vi "Parse Excel Doc.vi"(8 "error in (no error)":errorcluster, 11 "path":path) -> (0 "error out":errorcluster, 3 "Data":variant[][](array[variant]))   [LabVIEW 2019, in "Simple SysDef API.lvlib"]
uses:
  <userlib>/SimpleSysDef/Simple SysDef API.lvlib
panel:
  in  "Excel._Worksheet":refnum<k7>
  in  "Excel._Application":refnum<k7>
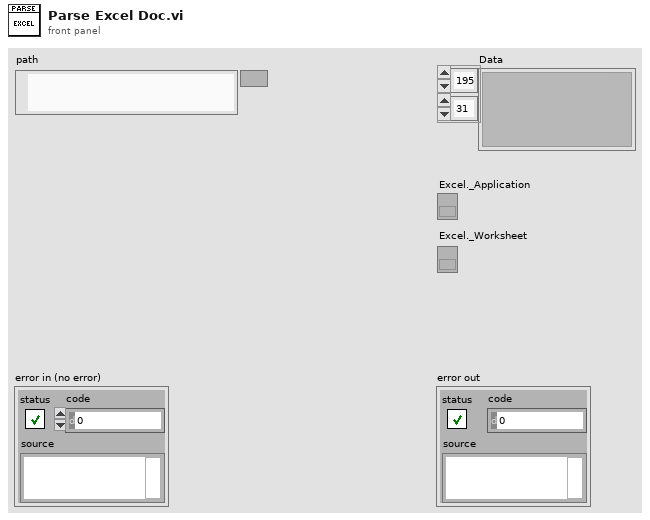
[diagram p1: front panel]
types:
  T1 = enum16{"maximized", "minimized", "normal", "no change"}
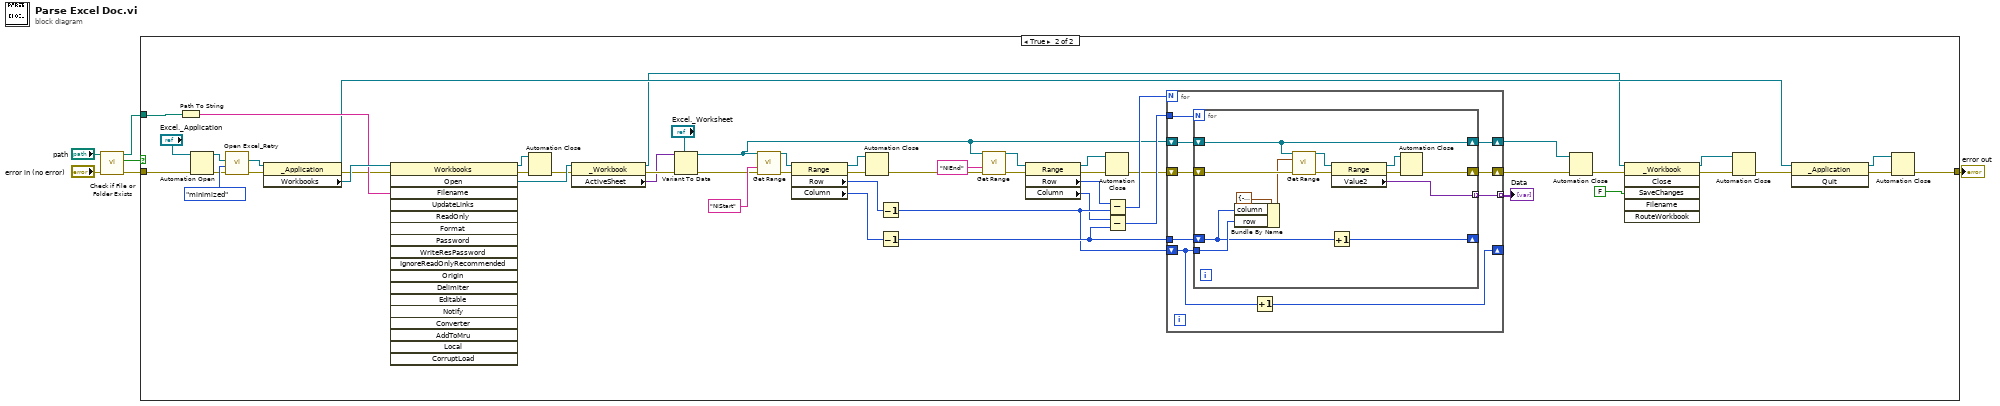
[diagram p0: block diagram]
diagram:
  n1 = call <vilib>:"Check if File or Folder Exists.vi"("error in (no error)"="error in (no error)", "path"="path") -> ("error out"=w5:errorcluster, "file or folder exists?"=w6:bool, "dup path"=w3:path)  [unwired: 7 in]
  n2 = case shown="True" w6 {
    tunnel: w5 -> [w7 w59]
    tunnel: w3 -> [_ w57]
    tunnel: [w7 w32] -> w2
    frame False {
    }
    frame True {
      n3 = Path To String(path=w57) -> (string=w56:string)
      n4 = Automation Open(error in (no error)=w59, Automation Refnum="Excel._Application") -> (Automation Refnum=w11:refnum<k7>, error out=w10:errorcluster)  [unwired: 1 in, 1 out]
      n5 = call <userlib>:"Open Excel_Retry.vi"("error in (no error)"=w10, "window state (normal)"=T1."minimized", "Excel._Application in"=w11) -> ("error out"=w9:errorcluster, "Excel._Application out"=w8:refnum<k7>)  [unwired: 7 in]
      n6 = property class="_Application"(reference=w8, error in=w9) -> (reference out=w28:refnum<k7>, error out=w42:errorcluster, "Workbooks"=w58:refnum<k7>)
      n7 = invoke class="Workbooks" method="Open"(reference=w58, error in=w42, "Filename"=w56) -> (reference out=w31:refnum<k7>, error out=w55:errorcluster, "Open"=w54:refnum<k7>)  [unwired: 15 in, 15 out]
      n8 = Automation Close(3:w55, 5:w31) -> (0:w53:errorcluster)
      n9 = property class="_Workbook"(reference=w54, error in=w53) -> (reference out=w26:refnum<k7>, error out=w51:errorcluster, "ActiveSheet"=w50:variant)
      n10 = Variant To Data(error in=w51, type="Excel._Worksheet", Variant=w50) -> (data=w17:refnum<k7>, error out=w20:errorcluster)
      n11 = call <userlib>:"Get Range.vi"("Excel._Worksheet"=w17, "name"="NIStart" ("name (\"\")"), "error in (no error)"=w20) -> ("Range"=w18:refnum<k7>, "error out"=w19:errorcluster)  [unwired: 11 in]
      n12 = property class="Range"(reference=w18, error in=w19) -> (reference out=w40:refnum<k7>, error out=w41:errorcluster, "Row"=w44:i32, "Column"=w38:i32)
      n13 = Automation Close(3:w41, 5:w40) -> (0:w13:errorcluster)
      n14 = Decrement(x=w44) -> (x-1=w43:i32)
      n15 = Decrement(x=w38) -> (x-1=w45:i32)
      n16 = call <userlib>:"Get Range.vi"("Excel._Worksheet"=w17, "name"="NIEnd" ("name (\"\")"), "error in (no error)"=w13) -> ("Range"=w16:refnum<k7>, "error out"=w15:errorcluster)  [unwired: 11 in]
      n17 = property class="Range"(reference=w16, error in=w15) -> (reference out=w35:refnum<k7>, error out=w37:errorcluster, "Row"=w48:i32, "Column"=w39:i32)
      n18 = Automation Close(3:w37, 5:w35) -> (0:w36:errorcluster)
      n19 = Subtract(x=w48, y=w43) -> (x-y=w47:i32)
      n20 = Subtract(x=w39, y=w45) -> (x-y=w46:i32)
      n21 = for {
        N: w47 -> [_]
        tunnel: w45 -> [w66]
        shift-right: [w64] -> _
        shift-left: w43 -> [w65]
        shift-right: [w68] -> w34
        shift-left: w36 -> [w69]
        tunnel: [w63] -> w49 mode=indexing
        tunnel: w46 -> [w62]
        shift-right: [w61] -> w33
        shift-left: w17 -> [w67]
        n22 = for {
          N: w62 -> [_]
          shift-right: [w76] -> w68
          shift-left: w69 -> [w74]
          tunnel: w65 -> [w81]
          shift-right: [w78] -> _
          shift-left: w66 -> [w79]
          tunnel: [w80] -> w63 mode=indexing
          shift-right: [w71] -> w61
          shift-left: w67 -> [w71]
          n23 = Bundle By Name(cluster=cluster{"row":i32, "column":i32} {"row"=-1, "column"=-1} ("start"), "column"=w79, "row"=w81) -> (w72:cluster{"row":i32, "column":i32})
          n24 = call <userlib>:"Get Range.vi"("Excel._Worksheet"=w71, "start"=w72, "error in (no error)"=w74) -> ("Range"=w70:refnum<k7>, "error out"=w73:errorcluster)  [unwired: 11 in]
          n25 = Increment(x=w79) -> (x+1=w78:i32)
          n26 = property class="Range"(reference=w70, error in=w73) -> (reference out=w75:refnum<k7>, error out=w77:errorcluster, "Value2"=w80:variant)
          n27 = Automation Close(3:w77, 5:w75) -> (0:w76:errorcluster)
        }
        n28 = Increment(x=w65) -> (x+1=w64:i32)
      }
      "Data" <- w49
      n29 = Automation Close(3:w34, 5:w33) -> (0:w25:errorcluster)
      n30 = invoke class="_Workbook" method="Close"(reference=w26, error in=w25, "SaveChanges"=FALSE) -> (reference out=w23:refnum<k7>, error out=w24:errorcluster)  [unwired: 3 in, 4 out]
      n31 = Automation Close(3:w24, 5:w23) -> (0:w30:errorcluster)
      n32 = invoke class="_Application" method="Quit"(reference=w28, error in=w30) -> (reference out=w27:refnum<k7>, error out=w29:errorcluster)  [unwired: 1 in, 1 out]
      n33 = Automation Close(3:w29, 5:w27) -> (0:w32:errorcluster)
    }
  }
  "error out" <- w2
